vi "CRYGet Weight Name Array for RTA.vi"() -> (3 "Weighting Names":string[](array[string]))   [LabVIEW 2013]
panel:
  in  "Weighting":string[](array[string])=["None", "A weighted", "B weighted", "C weighted", "ITU-R 468-4", "Dolby", "CCITT", "C-message", "Wb", "Wc", "Wd", "We", "Wf", "Wh", "Wj", "Wk", "Wm"]
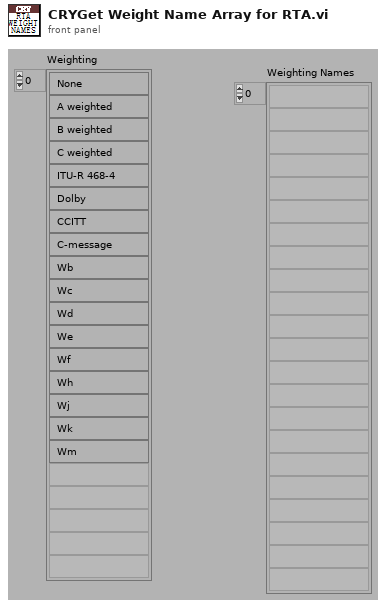
[diagram p1: front panel]
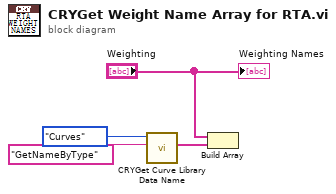
[diagram p0: block diagram]
diagram:
  n1 = call "CRYGet Curve Library Data Name.vi"("sAction"="GetNameByType", "Type"=enum16{"Curves", "Values", "Results", "WFM"}."Curves") -> ("sNames"=w2:string[])  [unwired: 6 in, 3 out]
  n2 = Build Array("Weighting", w2) -> ()  [unwired: 1 out]
  "Weighting Names" <- "Weighting"
